vi "TWM Client Cmd Set Corrections.vi"(4 "set digitizer (True)":bool=TRUE, 5 "timeout [ms]":i32=5000, 6 "set transducers (True)":bool, 7 "end of packet key":string="TWM:command:EndOfPacket", 8 "error in":errorcluster, 9 "digitizer correction":path, 10 "list of transducers":T1[](array[typedef]), 11 "handle":i32) -> (0 "error out":errorcluster, 3 "handle out":i32)   [LabVIEW 2020, in "TWM Client.lvlib"]
doc: "Write Set corrections command packet to TWM server. Wait for ACK. \"Set*\" flags must be set to actually send the command. Note the virtual channel indices in the transducer list are optional. Zero value means the low-side is disabled (single-ended mode). Zero value for high-side means the order of virtual channels will be generated automatically."
uses:
  TWM Client.lvlib
  TWM Client Transducer Correction Item.ctl
  1D I64.vi
  1D String.vi
  String.vi
  infolib.lvlib
panel:
  out "info data out":string
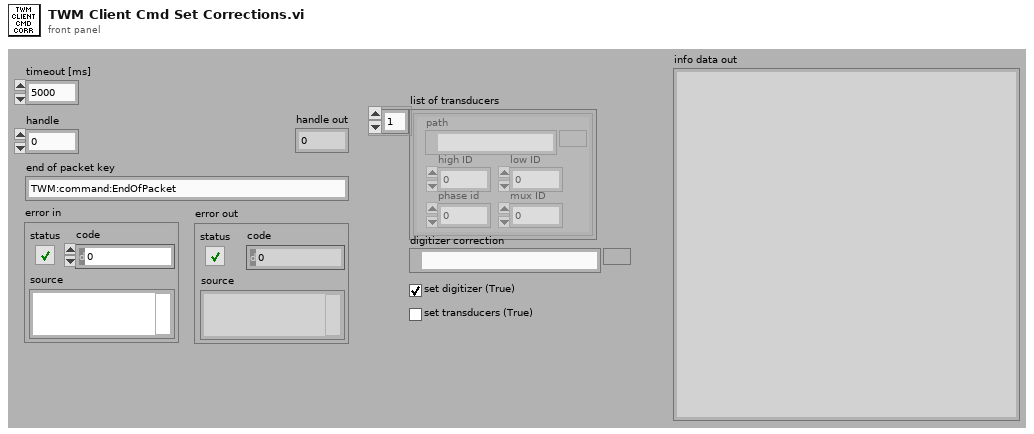
[diagram p1: front panel]
types:
  T1 = typedef "TWM Client.lvlib/TWM Client Transducer Correction Item.ctl" = cluster{"path":path, "high ID":i32, "low ID":i32, "phase id":i32, "mux ID":i32}
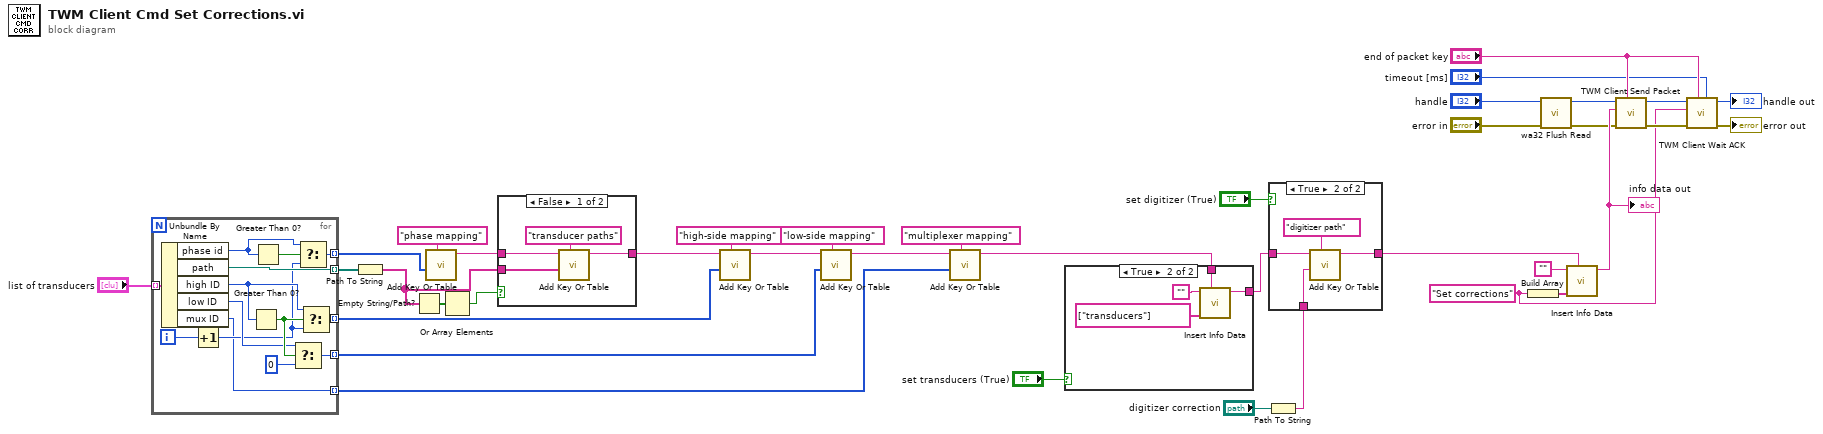
[diagram p0: block diagram]
diagram:
  w18 = "Set corrections" ("section name")
  n1 = for {
    tunnel: "list of transducers" -> [w52] mode=indexing
    tunnel: [w46] -> w9 mode=indexing
    tunnel: [w45] -> w36 mode=indexing
    tunnel: [w44] -> w33 mode=indexing
    tunnel: [w40] -> w13 mode=indexing
    tunnel: [w39] -> w11 mode=indexing
    i -> [w50]
    n2 = Unbundle By Name(w52) -> ("phase id"=w42:i32, "path"=w46:path, "high ID"=w51:i32, "low ID"=w48:i32, "mux ID"=w39:i32)
    n3 = Increment(x=w50) -> (x+1=w41:i32)
    n4 = Greater Than 0?(x=w51) -> (x > 0?=w49:bool)
    n5 = Greater Than 0?(x=w42) -> (x > 0?=w43:bool)
    n6 = Select(t=w48, s=w49, f=0) -> (s? t:f=w44:i32)
    n7 = Select(t=w42, s=w43, f=w41) -> (s? t:f=w40:i32)
    n8 = Select(t=w51, s=w49, f=w41) -> (s? t:f=w45:i32)
  }
  n9 = Path To String(path=w9) -> (string=w8:string[])
  n10 = Empty String/Path?(string/path=w8) -> (empty?=w7:bool[])
  n11 = call-poly "Add Key Or Table.vi"("key description"="phase mapping", "numeric"=w13) -> ("info data out"=w14:string)  [unwired: 8 in, 1 out]
  n12 = Or Array Elements(Boolean array=w7) -> (logical OR=w6:bool)
  n13 = case shown="False" w6 {
    tunnel: [w55 w57] -> w37
    tunnel: w14 -> [w54 w57]
    tunnel: w8 -> [w53 _]
    frame False {
      n14 = call-poly "Add Key Or Table.vi"("key description"="transducer paths", "string"=w53, "info data"=w54) -> ("info data out"=w55:string)  [unwired: 7 in, 1 out]
    }
    frame True {
    }
  }
  n15 = call-poly "Add Key Or Table.vi"("key description"="high-side mapping", "numeric"=w36, "info data"=w37) -> ("info data out"=w32:string)  [unwired: 7 in, 1 out]
  n16 = call-poly "Add Key Or Table.vi"("key description"="low-side mapping", "numeric"=w33, "info data"=w32) -> ("info data out"=w12:string)  [unwired: 7 in, 1 out]
  n17 = call-poly "Add Key Or Table.vi"("key description"="multiplexer mapping", "numeric"=w11, "info data"=w12) -> ("info data out"=w10:string)  [unwired: 7 in, 1 out]
  n18 = case shown="True" "set transducers (True)" {
    tunnel: w10 -> [_ w61]
    tunnel: [_ w59] -> w30
    frame False {
    }
    frame True {
      n19 = call "Insert Info Data.vi"("info data to insert"=w61, "sections"=string[] ["transducers"], "info data"="") -> ("info data out"=w59:string)  [unwired: 7 in, 1 out]
    }
  }
  n20 = Path To String(path="digitizer correction") -> (string=w27:string)
  n21 = case shown="True" "set digitizer (True)" {
    tunnel: w30 -> [w62 w66]
    tunnel: [w62 w64] -> w26
    tunnel: w27 -> [_ w63]
    frame False {
    }
    frame True {
      n22 = call-poly "Add Key Or Table.vi"("key description"="digitizer path", "string"=w63, "info data"=w66) -> ("info data out"=w64:string)  [unwired: 7 in, 1 out]
    }
  }
  n23 = Build Array(w18) -> (w24:string[])
  n24 = call "wa32 Flush Read.vi"("error in"="error in", "handle"="handle") -> ("error out"=w3:errorcluster, "handle out"=w2:i32)  [unwired: 7 in, 1 out]
  n25 = call "Insert Info Data.vi"("info data to insert"=w26, "sections"=w24, "info data"="") -> ("info data out"=w25:string)  [unwired: 7 in, 1 out]
  "info data out" <- w25
  n26 = call "TWM Client Send Packet.vi"("end of packet key"="end of packet key", "error in"=w3, "command string"=w25, "handle"=w2) -> ("error out"=w20:errorcluster, "handle out"=w17:i32)  [unwired: 6 in]
  n27 = call "TWM Client Wait ACK.vi"("timeout [ms] (3000)"="timeout [ms]", "key string"="end of packet key", "error in"=w20, "command header"=w18, "handle"=w17) -> ("error out"=→"error out":errorcluster, "handle out"=→"handle out":i32)  [unwired: 5 in]
